vi "eliascunha(frontpanel).vi"() -> ()   [LabVIEW 2020]
uses:
  <vilib>/LabVIEW Open Source Project/Epoch Date & Time/epoch.UNIX/Epoch.UNIX.lvclass
panel:
  in  "stop":bool
  out "Waveform Chart":waveform(dbl)(graph)
  out "output waveform":waveform(dbl)
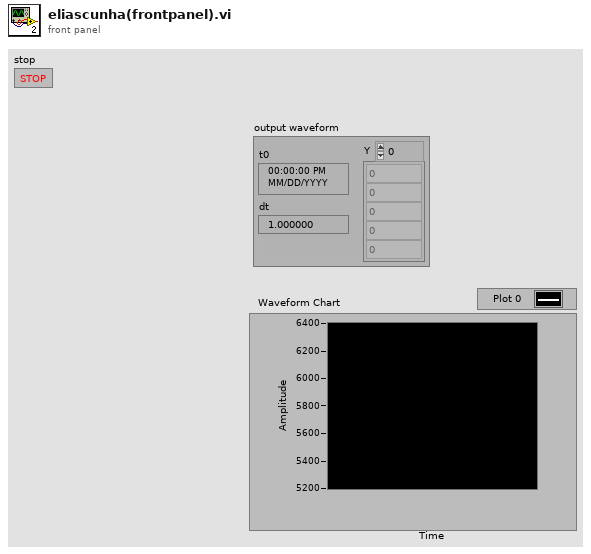
[diagram p1: front panel]
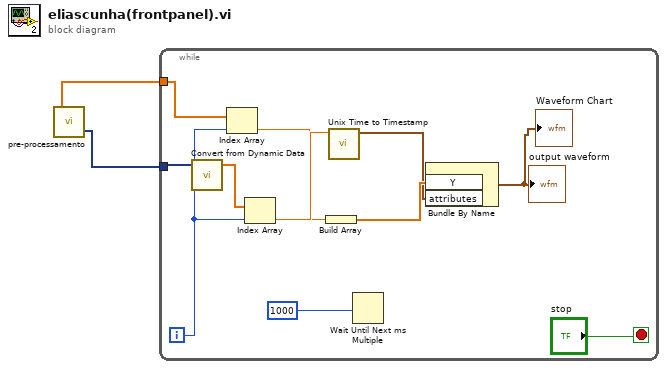
[diagram p0: block diagram]
diagram:
  n1 = call "pre-processamento.vi"() -> ("TimeStamp"=w1:dynamicdata, "Waveform Graph"=w2:dbl[])  [unwired: 2 out]
  n2 = while {
    tunnel: w2 -> [w13]
    tunnel: w1 -> [w12]
    i -> [w10]
    stop <- "stop" stop-if-true
    n3 = call "Convert from Dynamic Data"("Dynamic Data Type"=w12) -> ("Array"=w11:dbl[])  [unwired: 3 in]
    n4 = Index Array(array=w13, index=w10) -> (element=w3:dbl)
    n5 = Index Array(array=w11, index=w10) -> (element=w4:dbl)
    n6 = Build Array(w3) -> (w9:dbl[])
    n7 = call <vilib>:"Unix Time to Timestamp.vi"("Unix Time (s)"=w4) -> ("Timestamp"=w8:timestamp)  [unwired: 9 in, 1 out]
    n8 = Wait Until Next ms Multiple(millisecond multiple=u32 1000) -> ()  [unwired: 1 out]
    n9 = Bundle By Name("Y"=w9, "attributes"=w8) -> (→"output waveform" →"Waveform Chart":waveform(dbl))  [unwired: 1 in]
  }
